vi "cluster.vi"(0 "IMAGE PATH":path=path "C:/Users/swift/Desktop/Python/imec/Data/SKFX.300x300.Binning.2.frame.1.Gain.1.time.5.HDR-V3_corrected.hdr", 1 "Nb Iteration":i16=150, 4 "Nb Cluster":i16=4, 5 "ROI":T1) -> (7 "CENTRAL SPECTRA":dbl[][](array[numeric]), 8 "CLUSTERS":i32[][](array[numeric]))   [LabVIEW 2018]
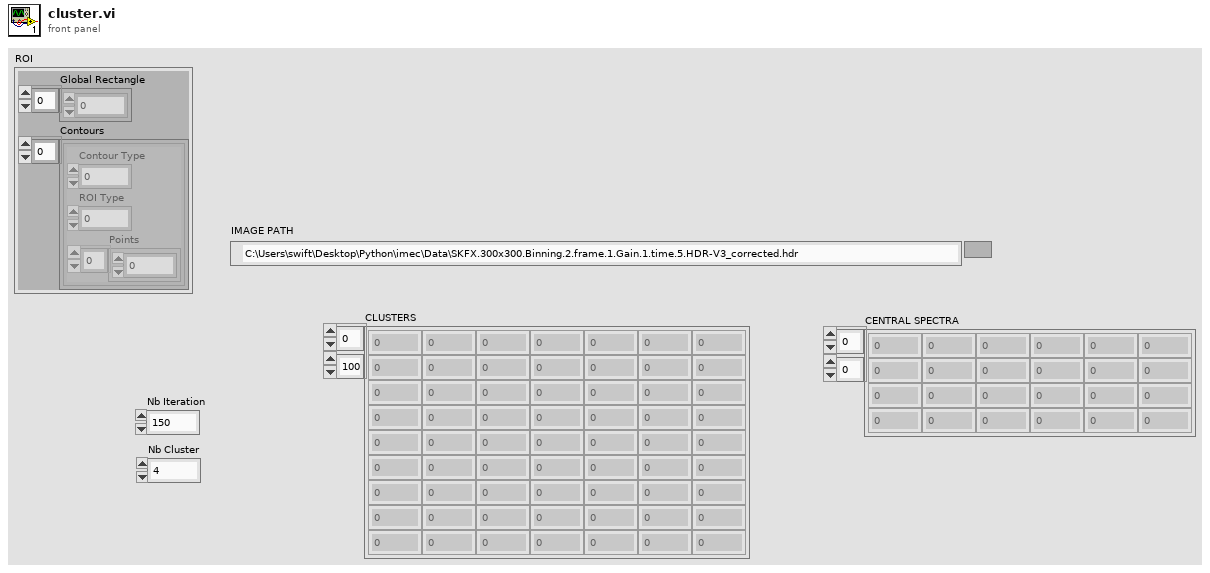
[diagram p1: front panel]
types:
  T1 = cluster{"Global Rectangle":i32[], "Contours":cluster{"Contour Type":u32, "ROI Type":u32, "Points":i32[]}[]}
  T2 = cluster{"Contour Type":u32, "ROI Type":u32, "Points":i32[]}[]
  T3 = cluster{"Contour Type":u32, "ROI Type":u32, "Points":i32[]}
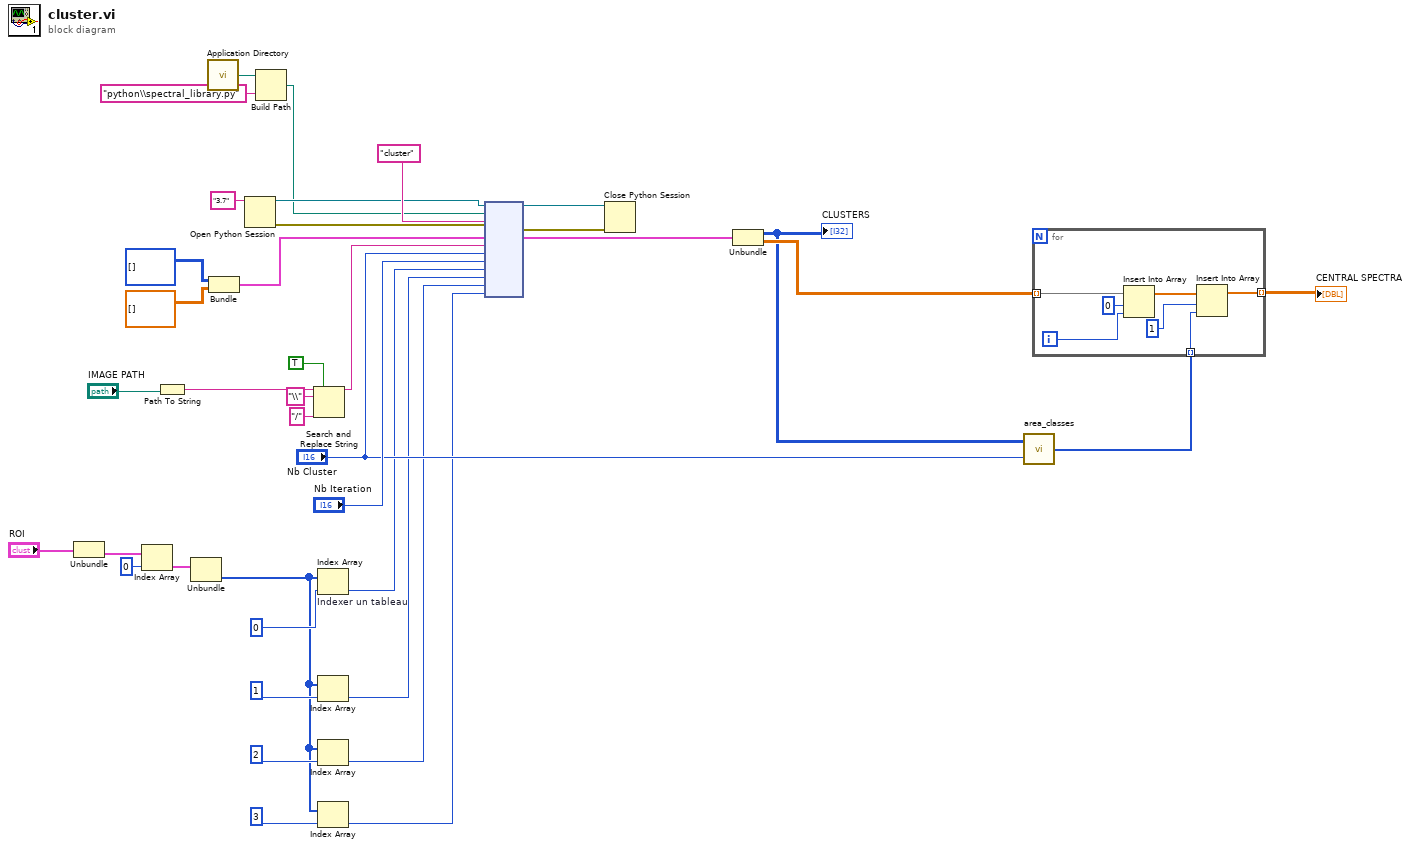
[diagram p0: block diagram]
diagram:
  n1 = Unbundle("ROI") -> ("Contours"=w13:T2)  [unwired: 1 out]
  n2 = Index Array(array=w13, index=0) -> (element=w11:T3)
  n3 = Path To String(path="IMAGE PATH") -> (string=w35:string)
  n4 = Unbundle(w11) -> ("Points"=w6:i32[])  [unwired: 2 out]
  n5 = call <vilib>:"Application Directory.vi"() -> ("Application Directory"=w26:path)
  n6 = Bundle(i32[][] [], dbl[][] []) -> (w20:cluster{i32[][], dbl[][]})  [unwired: 1 in]
  n7 = Open Python Session(python version="3.7" ("version Python")) -> (session out=w24:refnum<k35>, error out=w37:errorcluster)  [unwired: 2 in]
  n8 = Build Path(base path=w26, name or relative path="python\\spectral_library.py" ("nom ou chemin relatif")) -> (appended path=w23:path)
  n9 = Search and Replace String(replace all?=TRUE ("replace all? (F)"), input string=w35, search string="\\", replace string="/" ("replace string (\"\")")) -> (result string=w30:string)  [unwired: 4 in, 3 out]
  n10 = Index Array "Indexer un tableau"(array=w6, index=0 ("indice")) -> (element=w4:i32)
  n11 = Index Array(array=w6, index=1 ("indice")) -> (element=w3:i32)
  n12 = Index Array(array=w6, index=2 ("indice")) -> (element=w2:i32)
  n13 = Index Array(array=w6, index=3 ("indice")) -> (element=w1:i32)
  n14 = node(w24, w23, "cluster" ("nom de la fonction"), w37, w20, w30, "Nb Cluster", "Nb Iteration", w4, w3, w2, w1) -> (w28:refnum<k35>, w27:errorcluster, w19:cluster{i32[][], dbl[][]})  [unwired: 7 in, 2 out]
  n15 = Close Python Session(session in=w28, error in=w27) -> ()  [unwired: 1 out]
  n16 = Unbundle(w19) -> (w16:i32[][], w18:dbl[][])
  "CLUSTERS" <- w16
  n17 = call "area_classes.vi"("nb Class"="Nb Cluster", "CLUSTERS"=w16) -> ("Histogram: h(x)"=w17:i32[])
  n18 = for {
    tunnel: w18 -> [w45] mode=indexing
    tunnel: w17 -> [w40] mode=indexing
    tunnel: [w39] -> w14 mode=indexing
    i -> [w43]
    n19 = Insert Into Array(array=w45, index=0 ("indice"), new element=w43) -> (w42:dbl[])
    n20 = Insert Into Array(array=w42, index=1 ("indice"), new element=w40) -> (w39:dbl[])
  }
  "CENTRAL SPECTRA" <- w14
